vi "MD420_ACT_SetGradient.vi"(8 "error in":errorcluster, 9 "Gradient":dbl, 11 "MD420.lvclass in":refnum<class "MD420.lvclass">) -> (0 "error out":errorcluster, 3 "MD420.lvclass out":refnum<class "MD420.lvclass">)   [LabVIEW 2022 SP3]
uses:
  MD420.lvclass
  MD420.lvclass/MD420.ctl
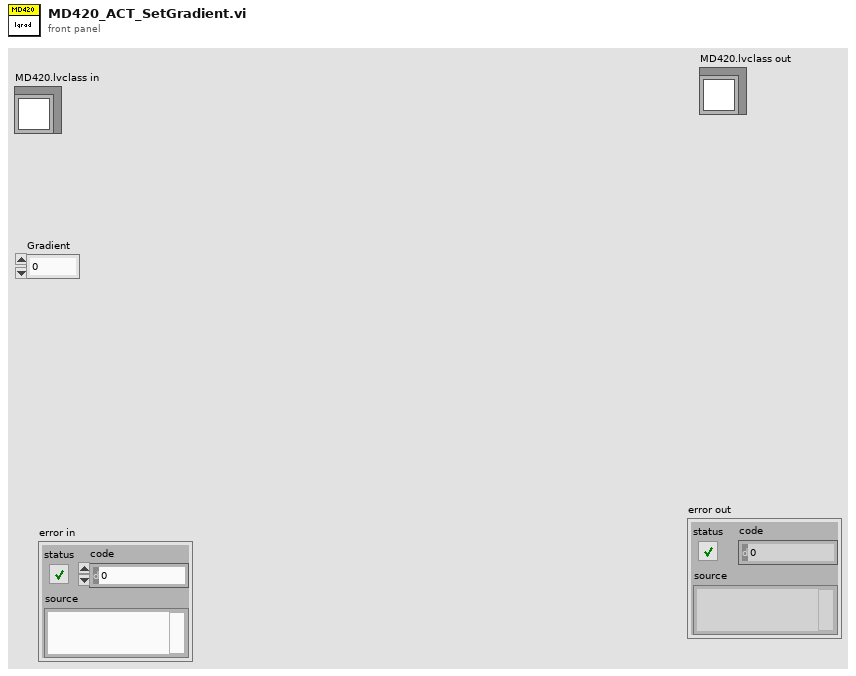
[diagram p1: front panel]
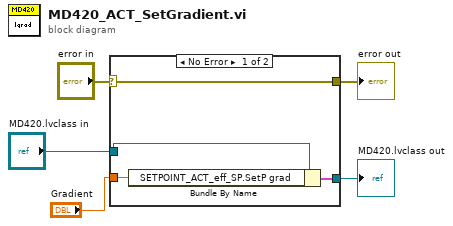
[diagram p0: block diagram]
diagram:
  n1 = case shown="No Error" "error in" {
    selector: "error in" -> [w6 w10]
    tunnel: "MD420.lvclass in" -> [w9 w11]
    tunnel: "Gradient" -> [w8 _]
    tunnel: [w7 w11] -> w2
    tunnel: [w6 w10] -> w1
    frame No Error {
      n2 = Bundle By Name(cluster=w9, "SETPOINT_ACT_eff_SP.SetP grad"=w8) -> (w7:cluster{})
    }
    frame Error {
    }
  }
  "error out" <- w1
  "MD420.lvclass out" <- w2
